vi "DAQ_Configure_ScanXY.vi"(6 "Continuous?":bool, 7 "Device name":string, 8 "error in":errorcluster caption="entrée d'erreur", 9 "2D Waveform":dbl[][](array[numeric]), 10 "N_Total":i32, 11 "Pixel_clock_Hz":dbl) -> (0 "error out":errorcluster caption="sortie d'erreur", 1 "AI task":refnum<k21>, 2 "AO task":refnum<k21>, 3 "CO task":refnum<k21>)   [LabVIEW 2026]
uses:
  <vilib>/DAQmx/write.llb/DAQmx Write (Analog 2D DBL NChan NSamp).vi
  <vilib>/DAQmx/create/channels.llb/DAQmx Create Channel (AO-Voltage-Basic).vi
  <vilib>/DAQmx/configure/timing.llb/DAQmx Timing (Sample Clock).vi
  <vilib>/DAQmx/miscellaneous.llb/DAQmx Fill In Error Info.vi
  <vilib>/DAQmx/create/channels.llb/DAQmx Create Channel (CO-Pulse Generation-Frequency).vi
  <vilib>/DAQmx/configure/timing.llb/DAQmx Timing (Implicit).vi
  <vilib>/DAQmx/create/channels.llb/DAQmx Create Channel (AI-Voltage-Basic).vi
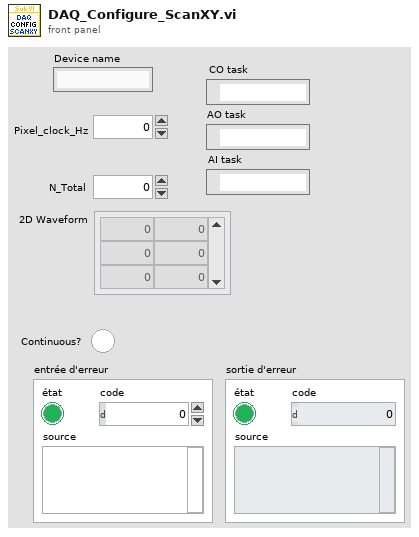
[diagram p1: front panel]
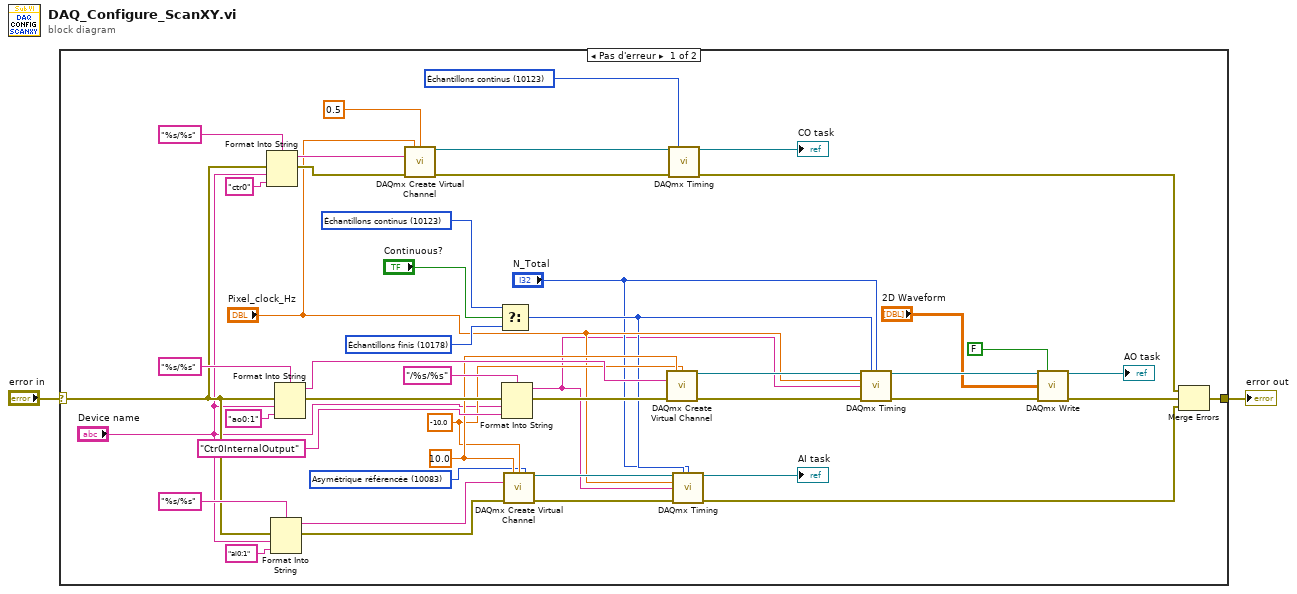
[diagram p0: block diagram]
diagram:
  n1 = case shown="Pas d'erreur" "error in" {
    selector: "error in" -> [w18 w49]
    tunnel: [w27 w49] -> w1
    frame No Error {
      w13 = 10083 items=["Par défaut"=-1, "Asymétrique référencée"=10083, "Asymétrique non référencée"=10078, "Différentielle"=10106, "Pseudodifférentielle"=12529] ("input terminal configuration")
      w33 = 10178 items=["Échantillons finis"=10178, "Échantillons continus"=10123, "Point par point avec cadencement matériel"=12522] ("sample mode")
      w34 = 10123 items=["Échantillons finis"=10178, "Échantillons continus"=10123, "Point par point avec cadencement matériel"=12522] ("sample mode")
      w14 = -10.0 ("minimum value")
      w15 = 10.0 ("maximum value")
      w41 = 10123 items=["Échantillons finis"=10178, "Échantillons continus"=10123, "Point par point avec cadencement matériel"=12522] ("sample mode")
      n2 = Format Into String(format string="%s/%s" ("chaîne de format"), error in=w18, "Device name", "ctr0" ("entrée 2")) -> (resulting string=w47:string, error out=w45:errorcluster)  [unwired: 1 in]
      n3 = Format Into String(format string="%s/%s" ("chaîne de format"), error in=w18, "Device name", "ai0:1" ("entrée 2")) -> (resulting string=w16:string, error out=w17:errorcluster)  [unwired: 1 in]
      n4 = Format Into String(format string="%s/%s" ("chaîne de format"), error in=w18, "Device name", "ao0:1" ("entrée 2")) -> (resulting string=w38:string, error out=w22:errorcluster)  [unwired: 1 in]
      n5 = call-poly <vilib>:"DAQmx Create Virtual Channel.vi"("frequency"="Pixel_clock_Hz", "duty cycle"=0.5, "counter"=w47, "error in"=w45) -> ("task out"=w42:refnum<k21>, "error out"=w43:errorcluster)  [unwired: 10 in]
      n6 = Select(t=w34, s="Continuous?", f=w33) -> (s? t:f=w9:i32)
      n7 = Format Into String(format string="/%s/%s" ("chaîne de format"), error in=w22, "Device name", "Ctr0InternalOutput" ("entrée 2")) -> (resulting string=w6:string, error out=w21:errorcluster)  [unwired: 1 in]
      n8 = call-poly <vilib>:"DAQmx Create Virtual Channel.vi"("maximum value"=w15, "minimum value"=w14, "input terminal configuration"=w13, "physical channels"=w16, "error in"=w17) -> ("task out"=w11:refnum<k21>, "error out"=w12:errorcluster)  [unwired: 9 in]
      n9 = call-poly <vilib>:"DAQmx Create Virtual Channel.vi"("maximum value"=w15, "minimum value"=w14, "physical channels"=w38, "error in"=w21) -> ("task out"=w36:refnum<k21>, "error out"=w37:errorcluster)  [unwired: 10 in]
      n10 = call-poly <vilib>:"DAQmx Timing.vi"("task/channels in"=w42, "sample mode"=w41, "error in"=w43) -> ("task out"=→"CO task":refnum<k21>, "error out"=w29:errorcluster)  [unwired: 11 in]
      n11 = call-poly <vilib>:"DAQmx Timing.vi"("task/channels in"=w11, "sample mode"=w9, "samples per channel"="N_Total", "rate"="Pixel_clock_Hz", "source"=w6, "error in"=w12) -> ("task out"=→"AI task":refnum<k21>, "error out"=w7:errorcluster)  [unwired: 8 in]
      n12 = call-poly <vilib>:"DAQmx Timing.vi"("task/channels in"=w36, "sample mode"=w9, "samples per channel"="N_Total", "rate"="Pixel_clock_Hz", "source"=w6, "error in"=w37) -> ("task out"=w31:refnum<k21>, "error out"=w32:errorcluster)  [unwired: 8 in]
      n13 = call-poly <vilib>:"DAQmx Write.vi"("task/channels in"=w31, "auto start"=FALSE, "data"="2D Waveform", "error in"=w32) -> ("task out"=→"AO task":refnum<k21>, "error out"=w28:errorcluster)  [unwired: 9 in, 1 out]
      n14 = Merge Errors(w29, w28, w7) -> (w27:errorcluster)
    }
    frame Error {
    }
  }
  "error out" <- w1
